vi "get_zoom_angle.vi"(8 "error in (no error)":errorcluster, 11 "TrajectoryMG100122AODFrameScan in":refnum<class "TrajectoryMG100122AODFrameScan.lvclass">) -> (0 "error out":errorcluster, 1 "z angle (phi)":dbl[unit], 2 "zoom":dbl, 3 "TrajectoryMG100122AODFrameScan out":refnum<class "TrajectoryMG100122AODFrameScan.lvclass">)   [LabVIEW 2010, in "TrajectoryMG100122AODFrameScan.lvclass"]
uses:
  TrajectoryMG100122AODFrameScan.lvclass
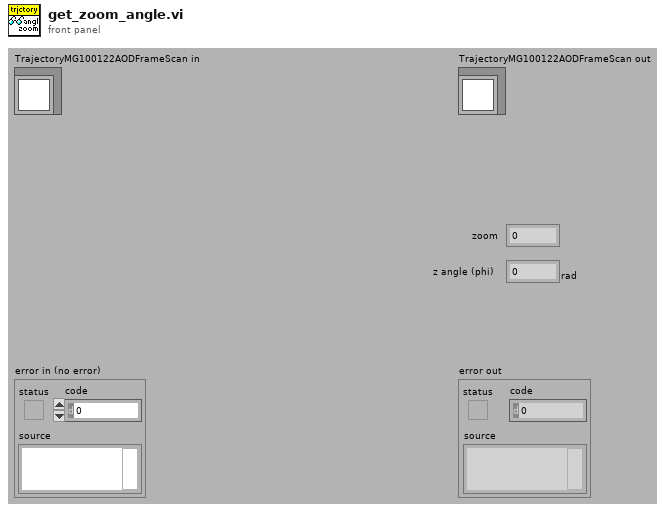
[diagram p1: front panel]
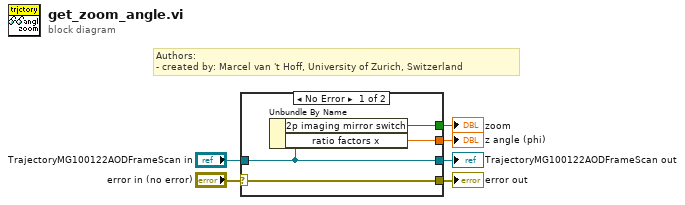
[diagram p0: block diagram]
diagram:
  # "Authors: \n- created by: Marcel van 't Hoff, University of Zurich, Switzerland"
  n1 = case shown="No Error" "error in (no error)" {
    selector: "error in (no error)" -> [w10 w11]
    tunnel: [w10 w11] -> w5
    tunnel: [w9 w12] -> w3
    tunnel: "TrajectoryMG100122AODFrameScan in" -> [w9 w12]
    tunnel: [w8 _] -> w2
    tunnel: [w7 _] -> w1
    frame No Error {
      n2 = Unbundle By Name(w9) -> ("2p imaging mirror switch"=w8:bool, "ratio factors x"=w7:dbl)
    }
    frame Error {
    }
  }
  "error out" <- w5
  "TrajectoryMG100122AODFrameScan out" <- w3
  "zoom" <- w2
  "z angle (phi)" <- w1
